vi "Flow_Globals.vi"() -> ()   [LabVIEW 2011]
panel:
  out "P Liquid Fow":dbl
  out "As Gas Flow":dbl
  out "P Gas Flow":dbl
  out "In Flow":dbl
  out "Ga 3 Flow":dbl
  out "Ga 2 Flow":dbl
  out "Ga 1 Flow":dbl
  out "Al Flow":dbl
  out "N2 Flow":dbl
  out "H2 Flow":dbl
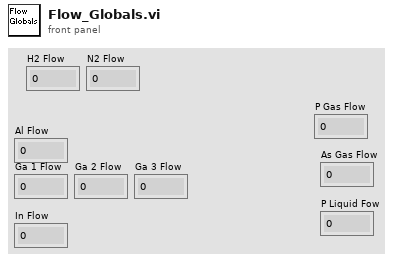
[diagram p1: front panel]
diagram:
